vi "ReadDataMK4.vi"(9 "millisecondIN":u32, 11 "input cluster":T1) -> (1 "millisecondOUT":u32, 2 "STATEUART":T3, 3 "Cluster":T2)   [LabVIEW 2017]
uses:
  mWorkToolkit/libSerial/STATEUART.ctl
  mWorkToolkit/libSerial/stateSerialUltra.ctl
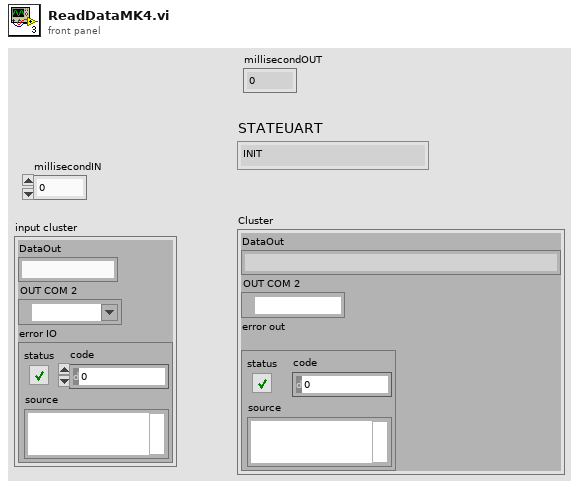
[diagram p1: front panel]
types:
  T1 = cluster{"DataOut":string, "OUT COM 2":refnum<visa-resource-name>, "error IO":errorcluster}
  T2 = cluster{"DataOut":string, "OUT COM 2":refnum<visa-resource-name>, "error out\n":errorcluster}
  T3 = typedef "STATEUART.ctl" = enum16{"INIT", "WRITE", "READ", "CHECKDATA", "IDLE", "STOP"}
  T4 = typedef "stateSerialUltra.ctl" = enum16{"findCOM", "Init", "CheckConnect", "Read", "Write", "exit"}
  T5 = cluster{"DataOut":string, "OUT COM 2":refnum<visa-resource-name>, "error out":errorcluster}
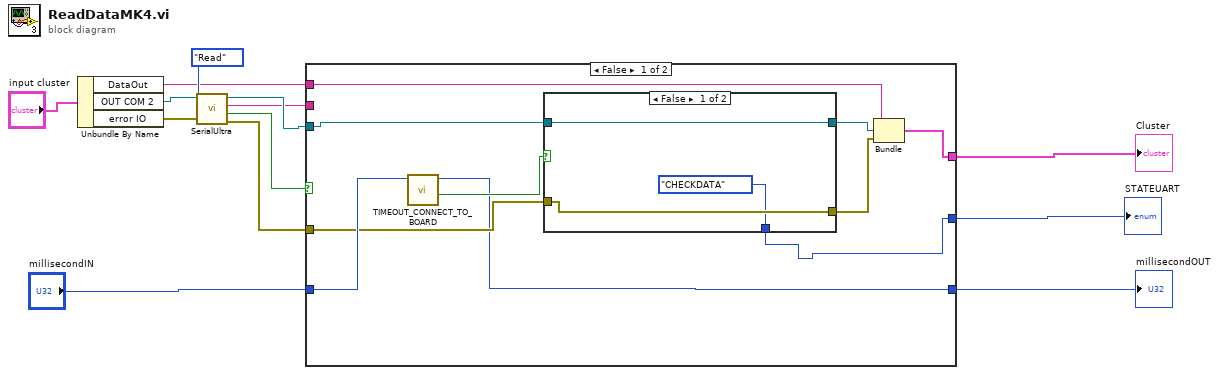
[diagram p0: block diagram]
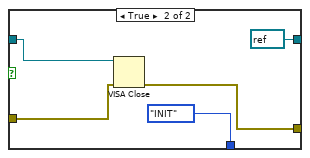
[diagram p2: hidden frame]
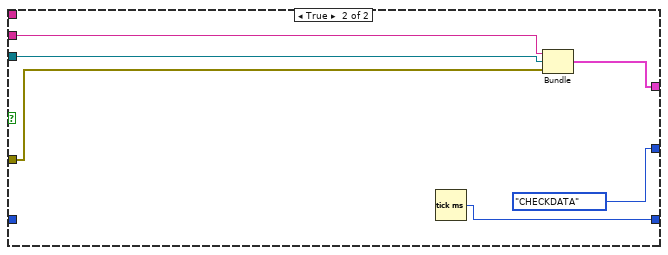
[diagram p3: hidden frame]
diagram:
  n1 = Unbundle By Name("input cluster") -> ("DataOut"=w1:string, "OUT COM 2"=w10:refnum<visa-resource-name>, "error IO"=w9:errorcluster)
  n2 = call "SerialUltra.vi"("error in"=w9, "State"=stateSerialUltra."Read", "IN COM"=w10) -> ("error out"=w11:errorcluster, "IsData"=w12:bool, "DataOut"=w7:string, "OUT COM 2"=w8:refnum<visa-resource-name>)  [unwired: 4 in, 1 out]
  n3 = case shown="False" w12 {
    tunnel: w11 -> [w21 w34]
    tunnel: "millisecondIN" -> [w23 _]
    tunnel: [w20 w37] -> w5
    tunnel: [w19 STATEUART."CHECKDATA"] -> w6
    tunnel: [w17 w33] -> w4
    tunnel: w8 -> [w18 w35]
    tunnel: w7 -> [_ w32]
    tunnel: w1 -> [w14 _]
    frame False {
      n4 = call "TIMEOUT_CONNECT_TO_BOARD.vi"("TIMEBEGIN"=w23) -> ("STATUS"=w22:bool, "TIMEOUT"=w20:u32)  [unwired: 9 in]
      n5 = case shown="False" w22 {
        tunnel: w18 -> [w24 w31]
        tunnel: w21 -> [w26 w30]
        tunnel: [w26 w29] -> w15
        tunnel: [STATEUART."CHECKDATA" STATEUART."INIT"] -> w19
        tunnel: [w24 refnum<visa-resource-name> refnum ("OUT COM 2")] -> w16
        frame False {
        }
        frame True {
          n6 = VISA Close(VISA resource name=w31, error in (no error)=w30) -> (error out=w29:errorcluster)
        }
      }
      n7 = Bundle("DataOut"=w14, "OUT COM 2"=w16, "error out"=w15) -> (w17:T5)  [unwired: 1 in]
    }
    frame True {
      n8 = Tick Count (ms)() -> (millisecond timer value=w37:u32)
      n9 = Bundle("DataOut"=w32, "OUT COM 2"=w35, "error out"=w34) -> (w33:T2)  [unwired: 1 in]
    }
  }
  "STATEUART" <- w6
  "millisecondOUT" <- w5
  "Cluster" <- w4
